vi "FTW-Container-Support-XML-CreateLVSchemaElement.vi"(0 "JSON Scalar Value":string, 5 "Node LV Type":string, 7 "Node Name":string, 11 "error in":errorcluster) -> (4 "LV Schema Node":string, 15 "error out":errorcluster)   [LabVIEW 2014, in "FTW-Container.lvclass"]
uses:
  FTW-Container.lvclass
panel:
  # "Inputs"
  # "Outputs"
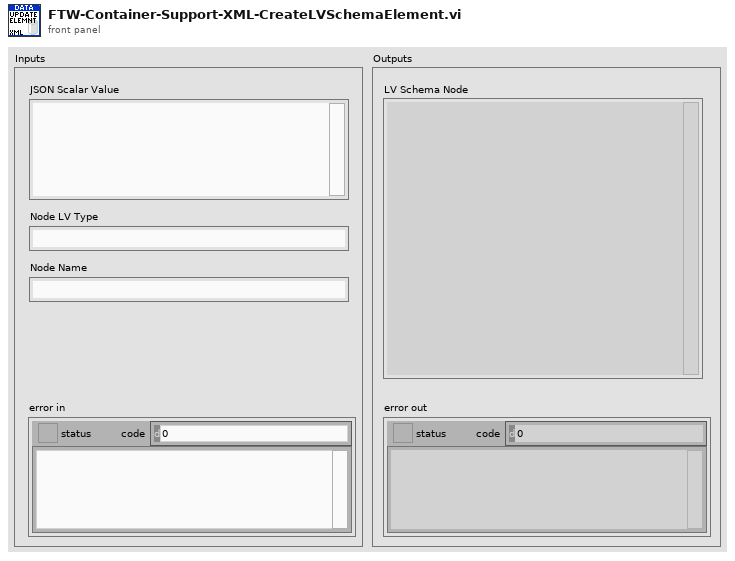
[diagram p1: front panel]
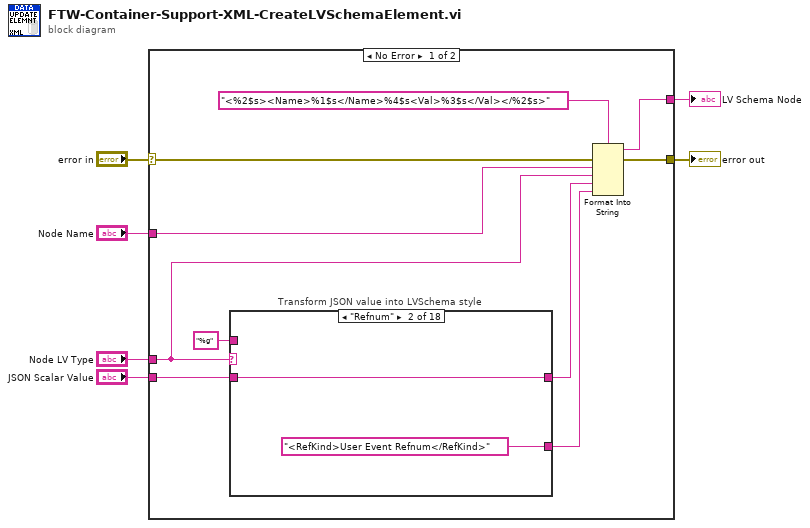
[diagram p0: block diagram]
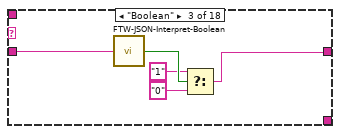
[diagram p3: hidden frame]
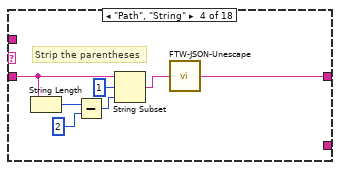
[diagram p4: hidden frame]
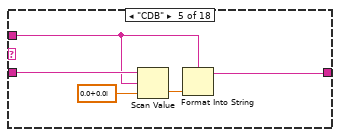
[diagram p5: hidden frame]
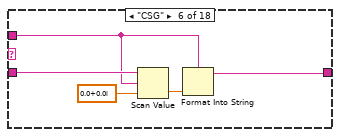
[diagram p6: hidden frame]
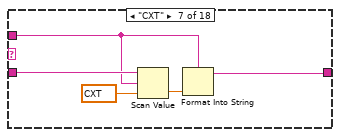
[diagram p7: hidden frame]
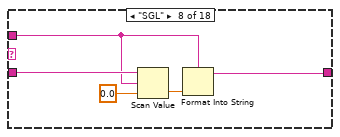
[diagram p8: hidden frame]
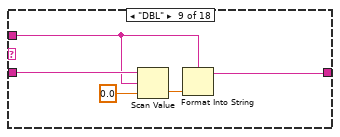
[diagram p9: hidden frame]
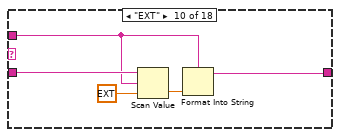
[diagram p10: hidden frame]
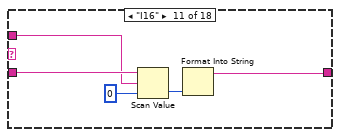
[diagram p11: hidden frame]
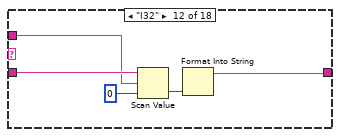
[diagram p12: hidden frame]
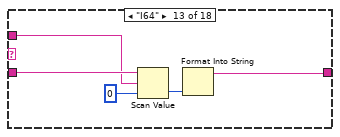
[diagram p13: hidden frame]
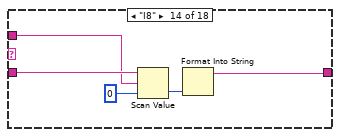
[diagram p14: hidden frame]
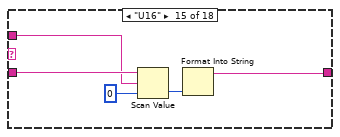
[diagram p15: hidden frame]
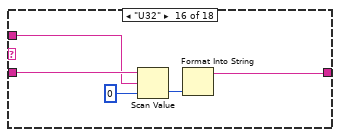
[diagram p16: hidden frame]
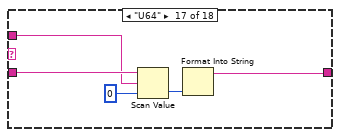
[diagram p17: hidden frame]
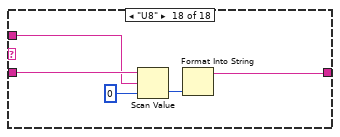
[diagram p18: hidden frame]
diagram:
  n1 = case shown="No Error" "error in" {
    selector: "error in" -> [w13 w102]
    tunnel: "JSON Scalar Value" -> [w16 _]
    tunnel: "Node LV Type" -> [w8 _]
    tunnel: [w10 w102] -> w4
    tunnel: "Node Name" -> [w15 _]
    tunnel: [w9 _] -> w1
    frame No Error {
      n2 = case "Transform JSON value into LVSchema style" shown="\"Refnum\"" w8 {
        tunnel: w16 -> [w17 w19 w21 w30 w36 w41 w46 w51 w56 w61 w66 w71 w76 w81 w86 w91 w96 w101]
        tunnel: [w17 w19 w20 w31 w33 w38 w43 w48 w53 w58 w63 w68 w73 w78 w83 w88 w93 w98] -> w14
        tunnel: "%g" ("format string") -> [_ _ _ _ w32 w37 w42 w47 w52 w57 w62 w67 w72 w77 w82 w87 w92 w97]
        tunnel: [_ "<RefKind>User Event Refnum</RefKind>" ("input 4") _ _ _ _ _ _ _ _ _ _ _ _ _ _ _ _] -> w7
        frame Default {
        }
        frame "Refnum" {
        }
        frame "Boolean" {
          n3 = call "FTW-JSON-Interpret-Boolean.vi"("JSON Boolean"=w21) -> ("LabVIEW Boolean"=w24:bool)
          n4 = Select(t="1", s=w24, f="0") -> (s? t:f=w20:string)
        }
        frame "Path", "String" {
          # "Strip the parentheses"
          n5 = String Length(string=w30) -> (length=w28:i32)
          n6 = Subtract(x=w28, y=2) -> (x-y=w27:i32)
          n7 = String Subset(string=w30, offset (0)=1, length (rest)=w27) -> (substring=w26:string)
          n8 = call "FTW-JSON-Unescape.vi"("Escaped UTF-8 String"=w26) -> ("Unescaped String"=w31:string)
        }
        frame "CDB" {
          n9 = Scan Value(string=w36, format string=w32, default (0 dbl)=cdb 0.0+0.0i) -> (value=w34:cdb)  [unwired: 1 out]
          n10 = Format Into String(format string=w32, w34) -> (resulting string=w33:string)  [unwired: 2 in, 1 out]
        }
        frame "CSG" {
          n11 = Scan Value(string=w41, format string=w37, default (0 dbl)=csg 0.0+0.0i) -> (value=w39:csg)  [unwired: 1 out]
          n12 = Format Into String(format string=w37, w39) -> (resulting string=w38:string)  [unwired: 2 in, 1 out]
        }
        frame "CXT" {
          n13 = Scan Value(string=w46, format string=w42, default (0 dbl)=cxt 0.0+0.0i) -> (value=w44:cxt)  [unwired: 1 out]
          n14 = Format Into String(format string=w42, w44) -> (resulting string=w43:string)  [unwired: 2 in, 1 out]
        }
        frame "SGL" {
          n15 = Scan Value(string=w51, format string=w47, default (0 dbl)=sgl 0.0) -> (value=w49:sgl)  [unwired: 1 out]
          n16 = Format Into String(format string=w47, w49) -> (resulting string=w48:string)  [unwired: 2 in, 1 out]
        }
        frame "DBL" {
          n17 = Scan Value(string=w56, format string=w52, default (0 dbl)=0.0) -> (value=w54:dbl)  [unwired: 1 out]
          n18 = Format Into String(format string=w52, w54) -> (resulting string=w53:string)  [unwired: 2 in, 1 out]
        }
        frame "EXT" {
          n19 = Scan Value(string=w61, format string=w57, default (0 dbl)=ext 0.0) -> (value=w59:ext)  [unwired: 1 out]
          n20 = Format Into String(format string=w57, w59) -> (resulting string=w58:string)  [unwired: 2 in, 1 out]
        }
        frame "I16" {
          n21 = Scan Value(string=w66, format string=w62, default (0 dbl)=i16 0) -> (value=w64:i16)  [unwired: 1 out]
          n22 = Format Into String(w64) -> (resulting string=w63:string)  [unwired: 3 in, 1 out]
        }
        frame "I32" {
          n23 = Scan Value(string=w71, format string=w67, default (0 dbl)=0) -> (value=w69:i32)  [unwired: 1 out]
          n24 = Format Into String(w69) -> (resulting string=w68:string)  [unwired: 3 in, 1 out]
        }
        frame "I64" {
          n25 = Scan Value(string=w76, format string=w72, default (0 dbl)=i64 0) -> (value=w74:i64)  [unwired: 1 out]
          n26 = Format Into String(w74) -> (resulting string=w73:string)  [unwired: 3 in, 1 out]
        }
        frame "I8" {
          n27 = Scan Value(string=w81, format string=w77, default (0 dbl)=i8 0) -> (value=w79:i8)  [unwired: 1 out]
          n28 = Format Into String(w79) -> (resulting string=w78:string)  [unwired: 3 in, 1 out]
        }
        frame "U16" {
          n29 = Scan Value(string=w86, format string=w82, default (0 dbl)=u16 0) -> (value=w84:u16)  [unwired: 1 out]
          n30 = Format Into String(w84) -> (resulting string=w83:string)  [unwired: 3 in, 1 out]
        }
        frame "U32" {
          n31 = Scan Value(string=w91, format string=w87, default (0 dbl)=u32 0) -> (value=w89:u32)  [unwired: 1 out]
          n32 = Format Into String(w89) -> (resulting string=w88:string)  [unwired: 3 in, 1 out]
        }
        frame "U64" {
          n33 = Scan Value(string=w96, format string=w92, default (0 dbl)=u64 0) -> (value=w94:u64)  [unwired: 1 out]
          n34 = Format Into String(w94) -> (resulting string=w93:string)  [unwired: 3 in, 1 out]
        }
        frame "U8" {
          n35 = Scan Value(string=w101, format string=w97, default (0 dbl)=u8 0) -> (value=w99:u8)  [unwired: 1 out]
          n36 = Format Into String(w99) -> (resulting string=w98:string)  [unwired: 3 in, 1 out]
        }
      }
      n37 = Format Into String(format string="<%2$s><Name>%1$s</Name>%4$s<Val>%3$s</Val></%2$s>", error in=w13, w15, w8, w14, w7) -> (resulting string=w9:string, error out=w10:errorcluster)  [unwired: 1 in]
    }
    frame Error {
    }
  }
  "error out" <- w4
  "LV Schema Node" <- w1
